vi "M01 Wind Turbine.vi"(11 "NXT/EV3":T1) -> (3 "EV3 out":T1)   [LabVIEW 2016]
uses:
  <vilib>/NXT/Subs/LVHSConnector.ctl
  <vilib>/NXT/LegoClasses/BrickReference/BrickReference.lvclass
  <vilib>/NXT/Block Support/NXT_InputPort.ctl
  <vilib>/NXT/Block Support/NXT_OutputPort.ctl
  <vilib>/NXT/NXTIO Xnodes/NXTIONodeSubVIs/NXTMotorRunDistance.vi
  <vilib>/NXT/NXTIO Xnodes/AddressXNode/NXTIOAddress.xnode
  <vilib>/NXT/NXTIO Xnodes/NXTIOXNode/NXTIO.xnode
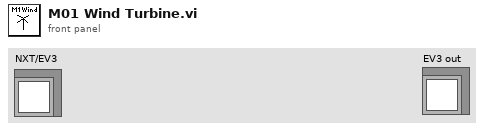
[diagram p1: front panel]
types:
  T1 = typedef "LVHSConnector.ctl" = refnum<class "BrickReference.lvclass">
  T2 = typedef "NXT_OutputPort.ctl" = u8
  T3 = typedef "NXT_InputPort.ctl" = u32
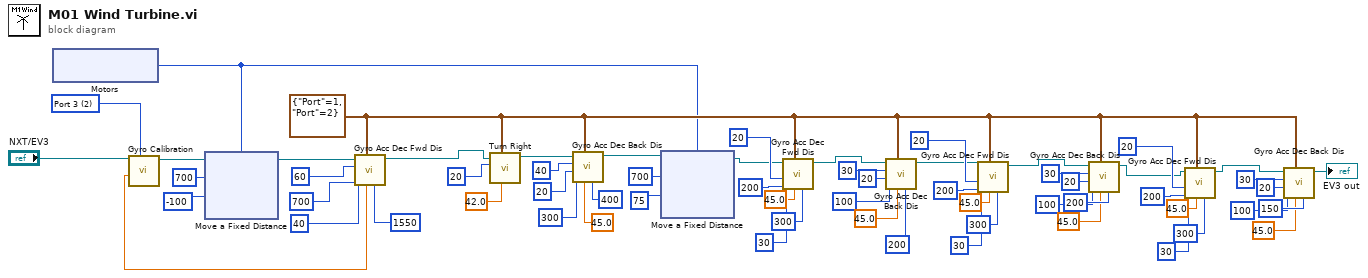
[diagram p0: block diagram]
diagram:
  w4 = cluster{"Port":T2, "Port":T2} {"Port"=1, "Port"=2} ("Motor")
  w62 = T3 2 items=["Port 1", "Port 2", "Port 3", "Port 4"] ("Port (Port 1)")
  n1 = xnode "Motors"() -> ("Motor"=w3:T2)
  n2 = call "Gyro Calibration.vi"("Port (Port 1)"=w62, "NXT/EV3"="NXT/EV3") -> ("Degrees"=w58:sgl, "NXT/EV3"=w61:T1)  [unwired: 5 in, 1 out]
  n3 = xnode "Move a Fixed Distance"("Speed 1"=i8 -100, "Distance 1"=700, "Motors"=w3, "NXT/EV3"=w61) -> ("NXT/EV3"=w5:T1)
  n4 = call "Gyro Acc Dec Fwd Dis.vi"("Stop rotation"=1550, "Ini. Degrees"=w58, "Motor"=w4, "Threshold to De-acc"=700, "De-acc"=40, "Acc"=60, "EV3 in"=w5) -> ("EV3 out"=w6:T1)  [unwired: 4 in]
  n5 = call "Turn Right.vi"("Turning angle"=sgl 42.0, "Motor"=w4, "Motor B (right)"=i8 20, "EV3 in"=w6) -> ("EV3 out"=w51:T1)  [unwired: 7 in]
  n6 = call "Gyro Acc Dec Back Dis.vi"("Stop rotation"=400, "Ini. Degrees"=sgl 45.0, "Motor"=w4, "Threshold to De-acc"=300, "De-acc"=20, "Acc"=40, "EV3 in"=w51) -> ("EV3 out"=w43:T1)  [unwired: 4 in]
  n7 = xnode "Move a Fixed Distance"("Speed 1"=i8 75, "Distance 1"=700, "Motors"=w3, "NXT/EV3"=w43) -> ("NXT/EV3"=w38:T1)
  n8 = call "Gyro Acc Dec Fwd Dis.vi"("Stop rotation"=300, "Ini. Degrees"=sgl 45.0, "Motor"=w4, "Threshold to De-acc"=200, "De-acc"=20, "Acc"=30, "EV3 in"=w38) -> ("EV3 out"=w31:T1)  [unwired: 4 in]
  n9 = call "Gyro Acc Dec Back Dis.vi"("Stop rotation"=200, "Ini. Degrees"=sgl 45.0, "Motor"=w4, "Threshold to De-acc"=100, "De-acc"=20, "Acc"=30, "EV3 in"=w31) -> ("EV3 out"=w19:T1)  [unwired: 4 in]
  n10 = call "Gyro Acc Dec Fwd Dis.vi"("Stop rotation"=300, "Ini. Degrees"=sgl 45.0, "Motor"=w4, "Threshold to De-acc"=200, "De-acc"=20, "Acc"=30, "EV3 in"=w19) -> ("EV3 out"=w30:T1)  [unwired: 4 in]
  n11 = call "Gyro Acc Dec Back Dis.vi"("Stop rotation"=200, "Ini. Degrees"=sgl 45.0, "Motor"=w4, "Threshold to De-acc"=100, "De-acc"=20, "Acc"=30, "EV3 in"=w30) -> ("EV3 out"=w7:T1)  [unwired: 4 in]
  n12 = call "Gyro Acc Dec Fwd Dis.vi"("Stop rotation"=300, "Ini. Degrees"=sgl 45.0, "Motor"=w4, "Threshold to De-acc"=200, "De-acc"=20, "Acc"=30, "EV3 in"=w7) -> ("EV3 out"=w18:T1)  [unwired: 4 in]
  n13 = call "Gyro Acc Dec Back Dis.vi"("Stop rotation"=150, "Ini. Degrees"=sgl 45.0, "Motor"=w4, "Threshold to De-acc"=100, "De-acc"=20, "Acc"=30, "EV3 in"=w18) -> ("EV3 out"=→"EV3 out":T1)  [unwired: 4 in]
